vi "USRP Throughput Streaming (FPGA).vi"() -> ()   [LabVIEW 2016]
doc: "Example Description:\nThis FPGA VI has two data streaming engines. One to stream data to disk from the FPGA and one to stream data from disk to the FPGA. The throughput of the streams is controled by accessing the DMA FIFOs on a subset of the cycles of the SCTLs.\n\nRunning the VI:\nThis VI m ust be run from one of the High Throughput Streaming - XXXXXXX (Host).vi files in the project. Refer to the host documentation for steps regarding running and configuring this FPGA VI.\n\nExecution Steps:\nRefer to teh block diagram of this VI for excution comments."
uses:
  <instrlib>/_niInstr/Register Bus/v1/FPGA/Public/Read Cmd Data.ctl
  <vilib>/Platform/TimedLoop/XDataNode/timing_clust.ctl
  <vilib>/Platform/TimedLoop/XDataNode/nitl_modes.ctl
  <vilib>/Platform/TimedLoop/XDataNode/wakeup.ctl
  <vilib>/rvi/Emulation/niFpgaSctlEmulationGetInTimedLoop.vi
  <vilib>/rvi/Emulation/niFpgaEmulationReportErrorSimple.vi
  <vilib>/rvi/Emulation/niFpgaGetClockAttributes.vi
  <vilib>/rvi/Emulation/niFpgaCriticalErrorInLSC.vi
  <vilib>/rvi/interface/RandomDataEmulation/nirviRandomDataMultiElementFPGAFIFO.vi
  <instcachedir>/0/nirviRandomDataMultiElementFPGAFIFO_6740B454F3C245F78F76ED91F73FD8DB.lvgen/nirviRandomDataMultiElementFPGAFIFO_6740B454F3C245F78F76ED91F73FD8DB_004.vi
  <vilib>/rvi/interface/RandomDataEmulation/niFpgaRandomDataHandleErrors.vi
  <vilib>/rvi/eio/common/nirviEmuTemplateMethod_errors.vi
  <vilib>/Platform/TimedLoop/XDataNode/XDataNode.xnode
  <vilib>/rvi/DataTransferAndStorage/Container/XNode/niFpgaContainer.xnode
  <vilib>/rvi/interface/RandomDataEmulation/nirviRandomDataFpgaMultiElementTemplate.vi
  <vilib>/eio/EIONode/EIONode.xnode
  <vilib>/Platform/TimedLoop/XDataNode/XDNodeRunTimeDep.lvlib
  <instrlib>/_niInstr/Register Bus/v1/FPGA/niInstr Register Bus v1 FPGA.lvlib
  <instrlib>/niUsrpRio/Config/v1/FPGA/niUsrpRio Config v1 FPGA.lvlib
panel:
  out "input.Max Throughput":u16
  out "output.Max Throughput":u16
  out "output.FIFO Size":u32
  out "input.FIFO Size":u32
  out "output.Ever Timed Out?":bool
  in  "output.Reset":bool
  out "output.Number of Elements to Read":u32
  out "output.Minimum Number of Elements to Read":u32
  out "output.FIFO Transfer Status":T1
  in  "output.Requested Throughput":u16
  in  "output.Requested Throughput Denominator":u16=200
  out "input.Ever Timed Out?":bool
  in  "input.Reset":bool
  out "input.Number of Elements to Write":u32
  out "input.Minimum Number of Elements to Write":u32
  out "input.FIFO Transfer Status":T2
  in  "input.Requested Throughput":u16
  in  "input.Requested Throughput Denominator":u16=200
  in  "reg.host read.go rcvd 0":bool
  out "reg.notify host.go 0":bool
  in  "reg.notify host.go rcvd 0":bool
  out "reg.host read.data 0":T3
  in  "reg.reset 0":bool
  in  "RF 0/Rx/Enable":bool
  in  "RF 0/Tx/Enable":bool
  in  "RF 1/Rx/Enable":bool
  in  "RF 1/Tx/Enable":bool
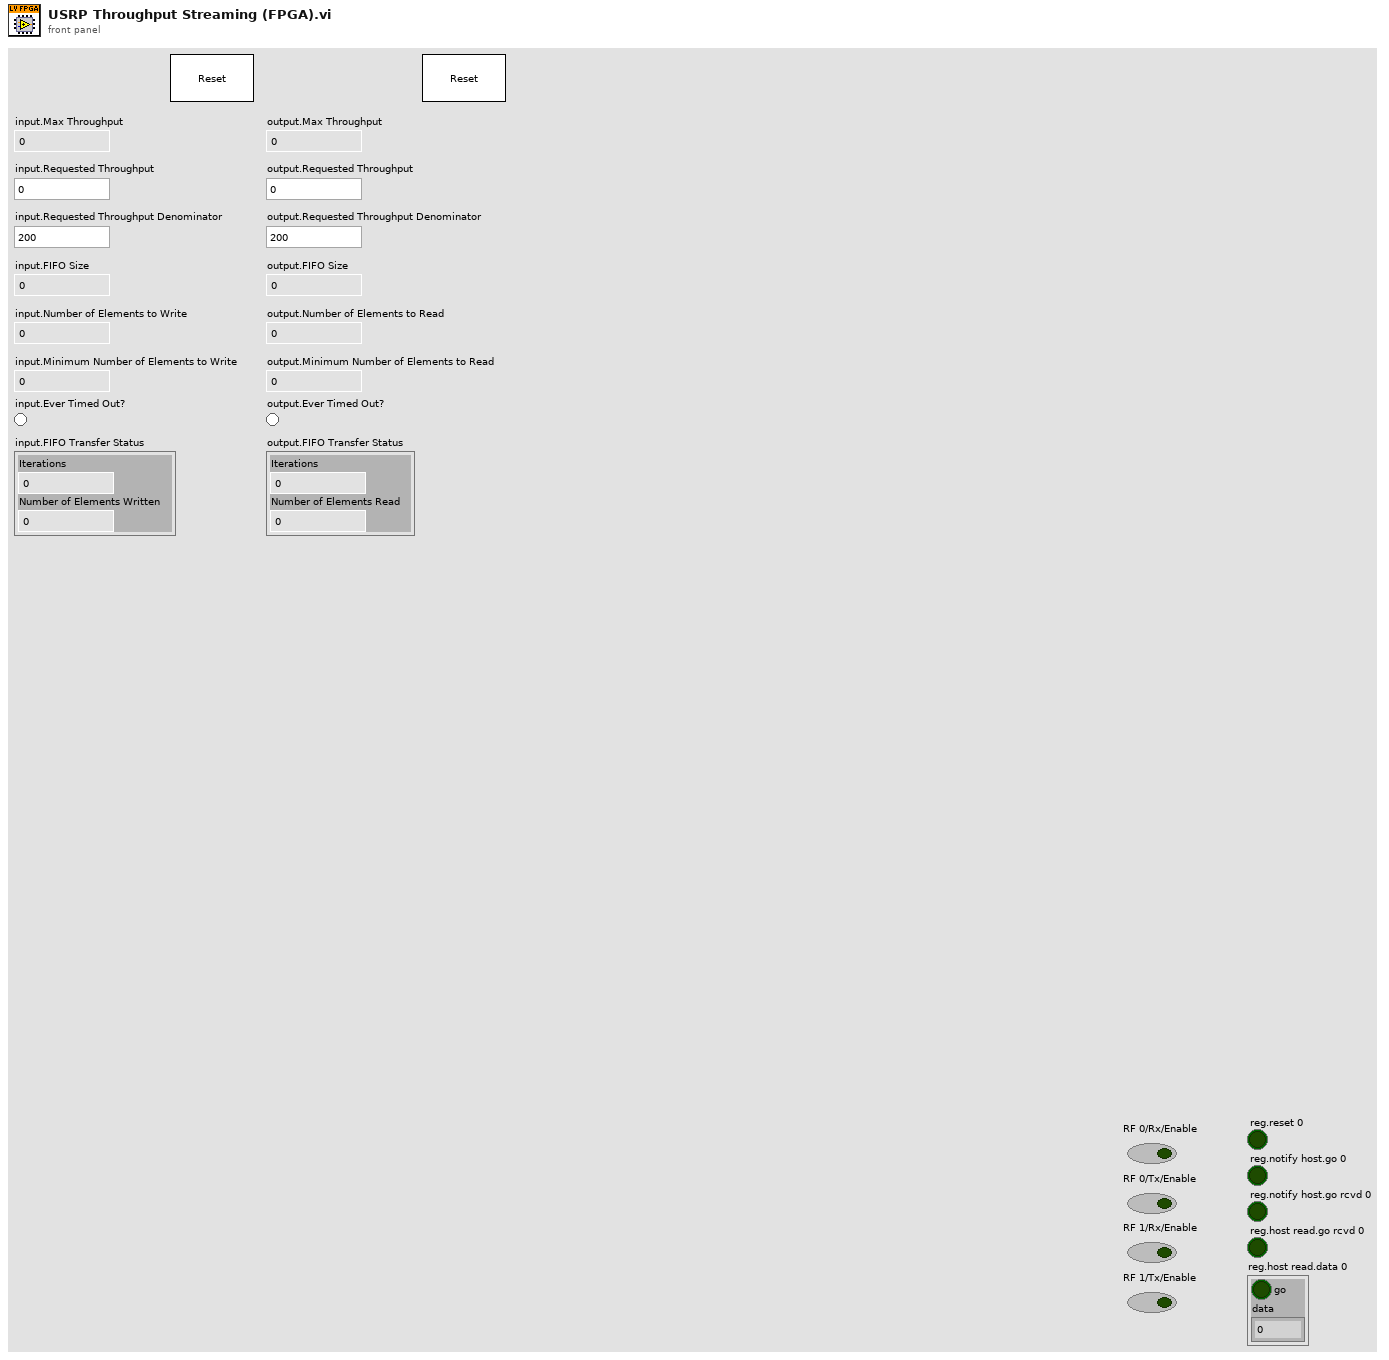
[diagram p1: front panel]
types:
  T1 = cluster{"Iterations":u64, "Number of Elements Read":u64}
  T2 = cluster{"Iterations":u64, "Number of Elements Written":u64}
  T3 = typedef "niInstr Register Bus v1 FPGA.lvlib/Read Cmd Data.ctl" = cluster{"go":bool, "data":u32}
  T4 = typedef "XDNodeRunTimeDep.lvlib/timing_clust.ctl" = cluster{"Expected End [f-1]":u64, "Actual End [f-1]":u64, "Finished Late? [f-1]":bool, "Expected End [i-1]":u64, "Actual End [i-1]":u64, "Finished Late? [i-1]":bool, "Expected Start [i]":u64, "Actual Start [i]":u64, "Expected Start [f]":u64, "Actual Start [f]":u64, "Source Name":string, "Structure Name":string, "Period":i64, "Deadline":i64, "Offset":i64, "Start":i64, "Priority":i32, "Timeout":i32, "Mode":T5, "Wakeup Reason":T6, "Error":errorcluster, "Source Type":string, "Secondary Source Type":string, "Global End Time":u64, "Global Start Time":u64, "Frame Duration":u64, "Iteration Duration":u64, "Assigned CPU":i32, "I/O Scan Engine Mode":u32}
  T5 = typedef "XDNodeRunTimeDep.lvlib/nitl_modes.ctl" = enum32{"No Change", "Process missed periods, maintain original phase", "Discard missed periods, maintain original phase", "Process missed periods, ignore original phase", "Discard missed periods, ignore original phase"}
  T6 = typedef "XDNodeRunTimeDep.lvlib/wakeup.ctl" = enum32{"Normal", "Aborted", "Asynchronous wakeup", "Timing source error", "Timed loop error", "Timeout"}
  T7 = cluster{"DAC FIFO Reset":refnum<k21>, "RF 0 Rx Swap IQ":refnum<k21>, "RF 0 Rx Negate I":refnum<k21>, "RF 0 Rx Negate Q":refnum<k21>, "RF 0 Rx Data Valid":refnum<k21>, "RF 0 Rx Data Ever Invalid":refnum<k21>, "clear RF 0 Rx Data Ever Invalid":refnum<k21>, "RF 0 Tx Swap IQ":refnum<k21>, "RF 0 Tx Negate I":refnum<k21>, "RF 0 Tx Negate Q":refnum<k21>, "RF 1 Rx Swap IQ":refnum<k21>, "RF 1 Rx Negate I":refnum<k21>, "RF 1 Rx Negate Q":refnum<k21>, "RF 1 Rx Data Valid":refnum<k21>, "RF 1 Rx Data Ever Invalid":refnum<k21>, "clear RF 1 Rx Data Ever Invalid":refnum<k21>, "RF 1 Tx Swap IQ":refnum<k21>, "RF 1 Tx Negate I":refnum<k21>, "RF 1 Tx Negate Q":refnum<k21>}
  T8 = typedef "niUsrpRio Synchronization v1 FPGA.lvlib/Resources.ctl" = cluster{"master":refnum<k21>, "meas.enable":refnum<k21>, "meas.ready":refnum<k21>, "meas.reset":refnum<k21>, "meas.arm":refnum<k21>, "meas.valid":refnum<k21>, "meas.value":refnum<k21>, "meas.oversample factor":refnum<k21>, "cptr":refnum<k21>, "cptr.adjust":refnum<k21>, "cptr.period":refnum<k21>}
  T9 = typedef "niUsrpRio Time v1 FPGA.lvlib/Time Resources.ctl" = cluster{"reset":refnum<k21>, "time":refnum<k21>, "time.previous cptr":refnum<k21>, "new time":refnum<k21>, "new time.when":refnum<k21>, "new time.set":refnum<k21>, "which edge of ref":refnum<k21>, "pps source":refnum<k21>, "internal pps period":refnum<k21>}
  T10 = typedef "niUsrpRio Time v1 FPGA.lvlib/Future Event Resources.ctl" = cluster{"reset":refnum<k21>, "future event.time":refnum<k21>, "future event.ready":refnum<k21>, "future event.set":refnum<k21>, "future event.clear":refnum<k21>, "future event.set in past":refnum<k21>}
  T11 = cluster{"time.resources":T9, "future event.resources":T10, "future event.resources":T10, "future event.resources":T10}
  T12 = typedef "niInstr Register Bus v1 FPGA.lvlib/Register Instruction.ctl" = cluster{"subsystem":u8, "address":u16, "data":u32, "valid":bool, "read":bool}
  T13 = typedef "niInstr Register Bus v1 FPGA.lvlib/Read Completion.ctl" = cluster{"data":u32, "valid":bool}
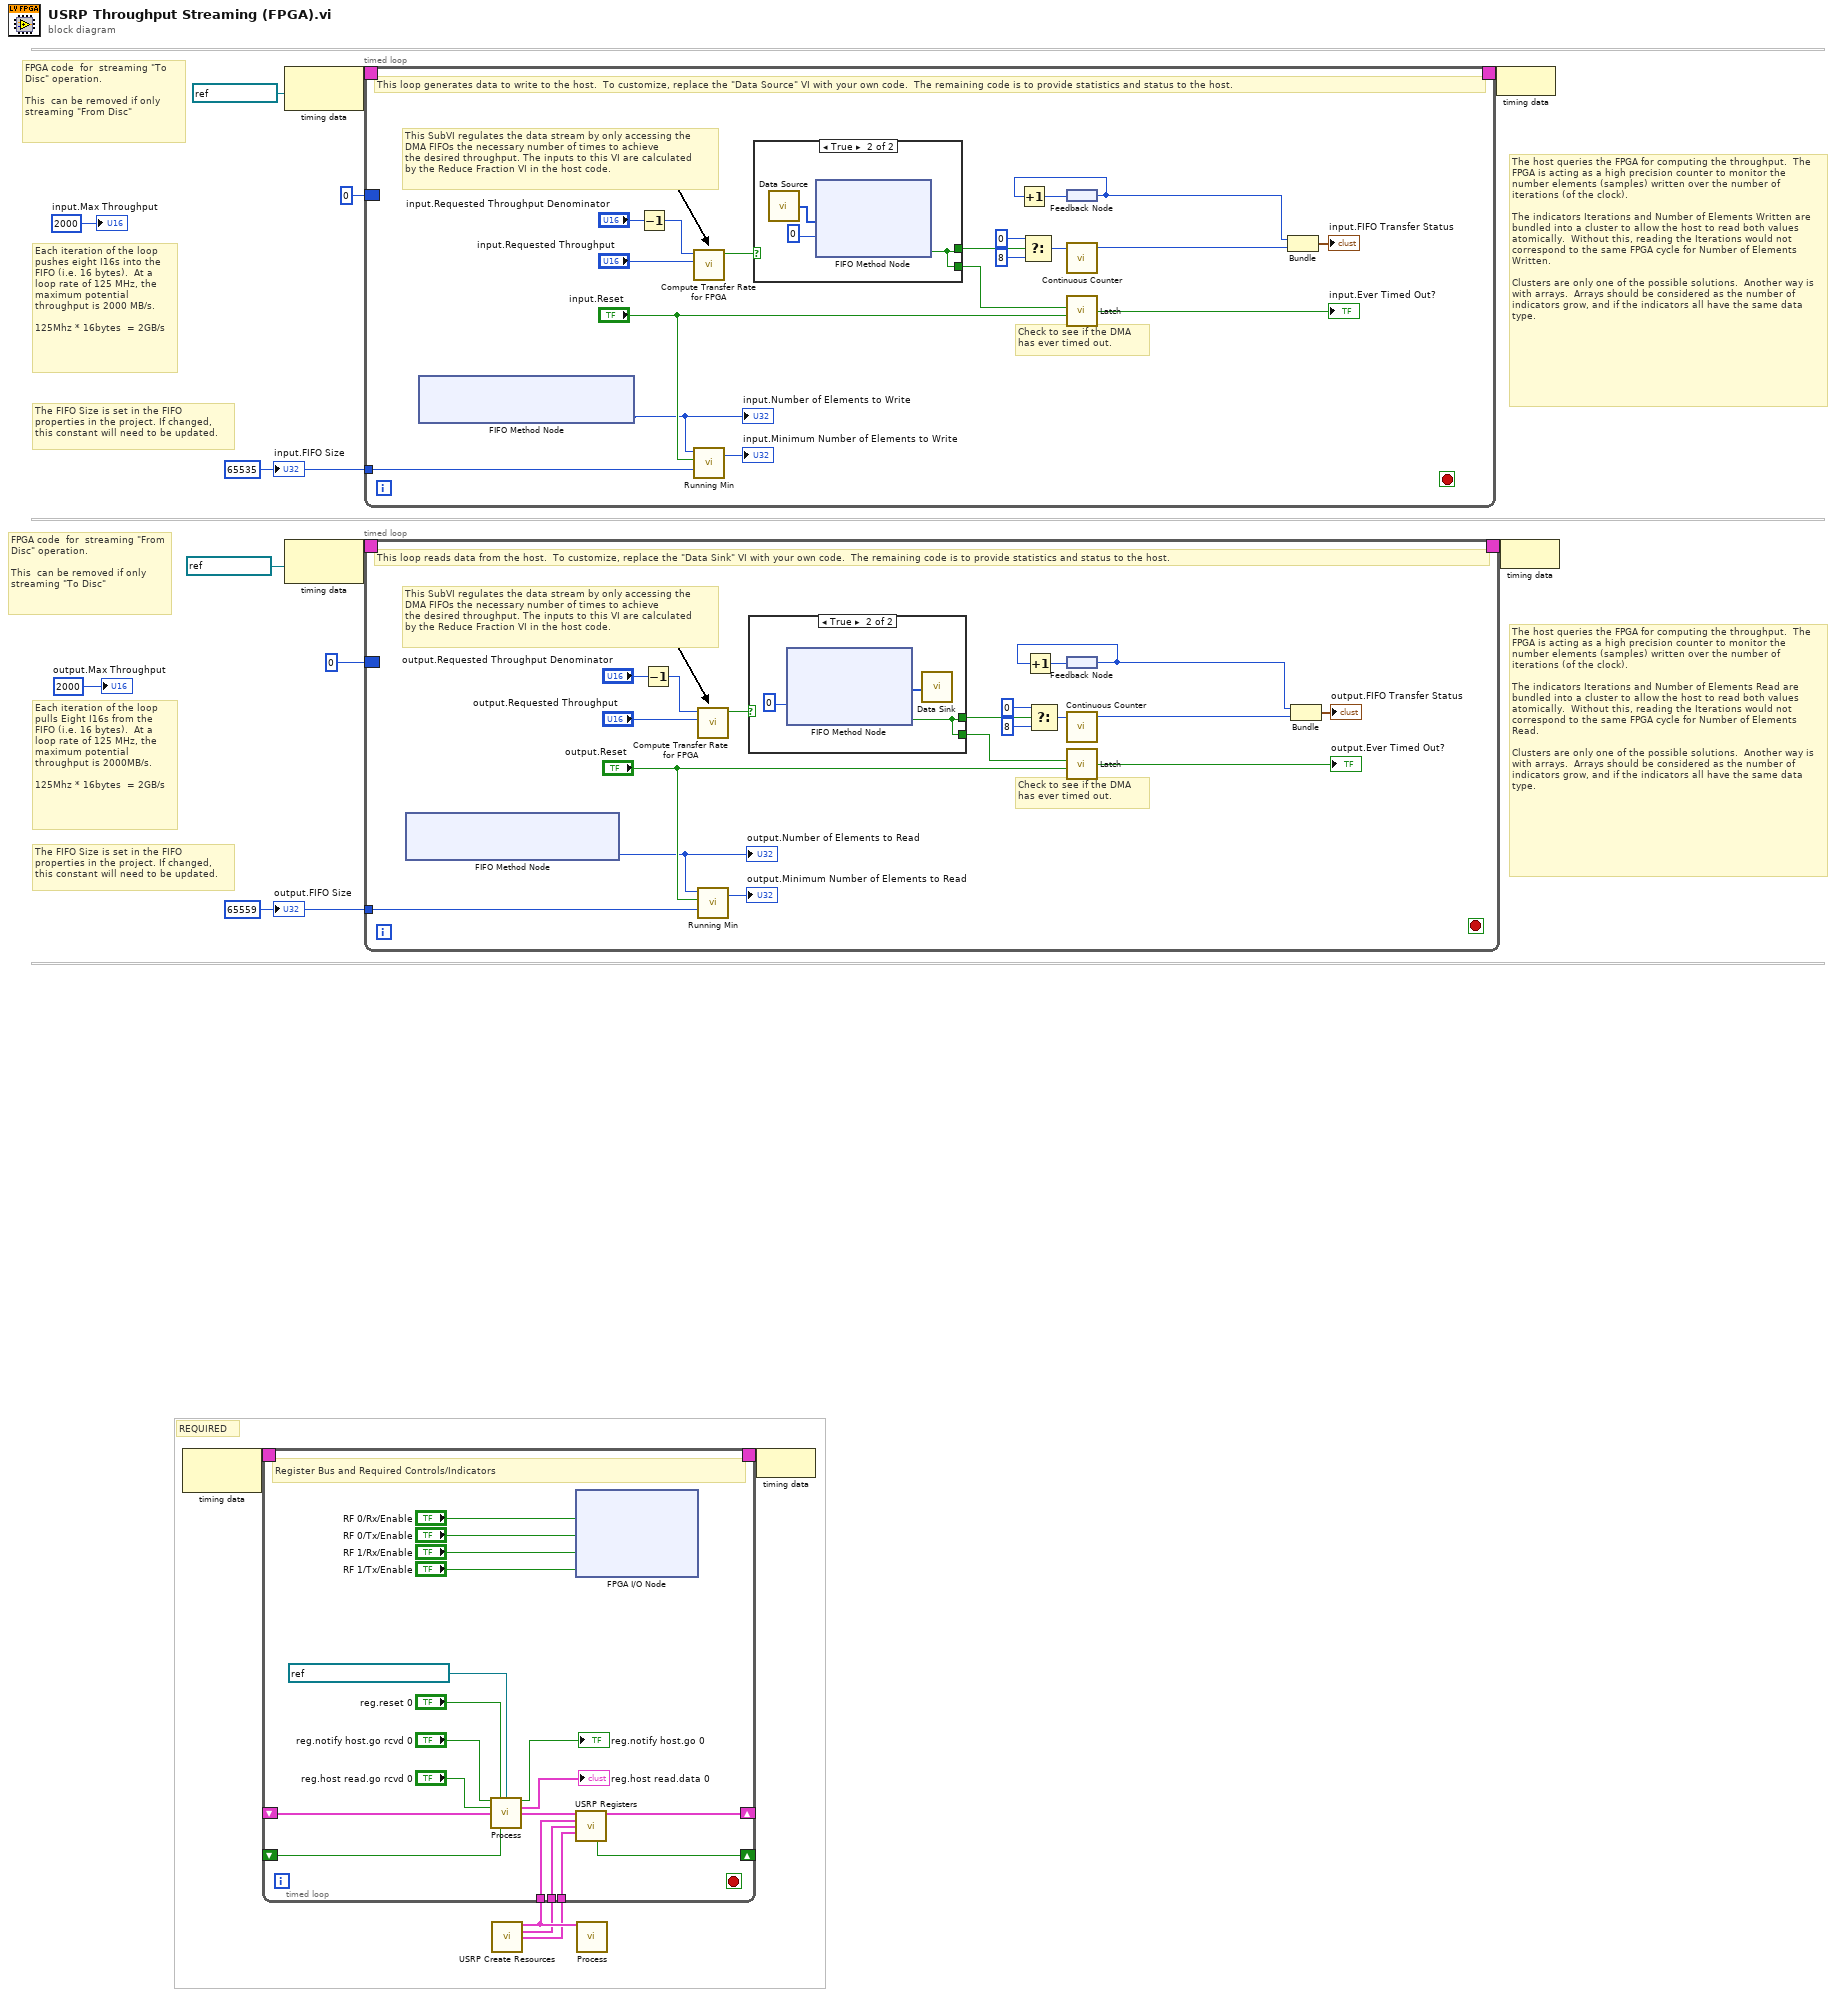
[diagram p0: block diagram]
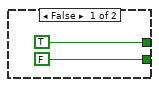
[diagram p2: hidden frame]
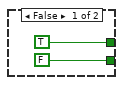
[diagram p3: hidden frame]
diagram:
  w6 = u32 65559 ("output.FIFO Size")
  w3 = u32 65535 ("input.FIFO Size")
  # "The FIFO Size is set in the FIFO\nproperties in the project. If changed, \nthis constant will need to be updated."
  # "The FIFO Size is set in the FIFO\nproperties in the project. If changed, \nthis constant will need to be updated."
  # "FPGA code  for  streaming \"To Disc\" operation. \n\nThis  can be removed if only streaming \"From Disc\""
  # "FPGA code  for  streaming \"From Disc\" operation. \n\nThis  can be removed if only streaming \"To Disc\""
  # "Each iteration of the loop pulls Eight I16s from the FIFO (i.e. 16 bytes).  At a loop rate of 125 MHz, the maximum potential throughput is 2000MB/s.\n\n125Mhz * 16bytes  = 2GB/s"
  # "The host queries the FPGA for computing the throughput.  The FPGA is acting as a high precision counter to monitor the number elements (samples) written over the number of iterations (of the clock).\n\nThe indicators Iterations and Number of Elements Read are bundled into a cluster to allow the host to read both values atomically.  Without this, reading the Iterations would not correspond to the same FPGA cycle for Number of Elements Read.\n\nClusters are only one of the possible solutions.  Another way is with arrays.  Arrays should be considered as the number of indicators grow, and if the indicators all have the same data type."
  # "Each iteration of the loop pushes eight I16s into the FIFO (i.e. 16 bytes).  At a loop rate of 125 MHz, the maximum potential throughput is 2000 MB/s.\n\n125Mhz * 16bytes  = 2GB/s"
  # "The host queries the FPGA for computing the throughput.  The FPGA is acting as a high precision counter to monitor the number elements (samples) written over the number of iterations (of the clock).\n\nThe indicators Iterations and Number of Elements Written are bundled into a cluster to allow the host to read both values atomically.  Without this, reading the Iterations would not correspond to the same FPGA cycle for Number of Elements Written.\n\nClusters are only one of the possible solutions.  Another way is with arrays.  Arrays should be considered as the number of indicators grow, and if the indicators all have the same data type."
  # "REQUIRED"
  n1 = node-c288() -> (w17:T4)  [unwired: 1 in]
  n2 = node-c288(refnum<k21> "Data Clock" ("Source Name")) -> (w12:T4)
  n3 = node-c288(refnum<k21> "Data Clock" ("Source Name")) -> (w10:T4)
  n4 = timed-loop {
    timing: w12 -> [_]
    timing-out: [_] -> w11
    tunnel: w3 -> [w35]
    border: u64 0 -> [_]
    stop <- _ stop-if-true
    # "Check to see if the DMA \nhas ever timed out."
    # "This SubVI regulates the data stream by only accessing the \nDMA FIFOs the necessary number of times to achieve \nthe desired throughput. The inputs to this VI are calculated \nby the Reduce Fraction VI in the host code."
    # "This loop generates data to write to the host.  To customize, replace the \"Data Source\" VI with your own code.  The remaining code is to provide statistics and status to the host."
    n5 = xnode ("FIFO Method Node")() -> ("Number of Elements to Write"=w18:u32)  [unwired: 1 in, 1 out]
    "input.Number of Elements to Write" <- w18
    n6 = Decrement(x="input.Requested Throughput Denominator") -> (x-1=w20:u16)
    n7 = call "Compute Transfer Rate for FPGA.vi"("Duty Rate"="input.Requested Throughput", "Clock Rate (minus 1)"=w20) -> ("Output"=w23:bool)  [unwired: 4 in, 1 out]
    n8 = call "Running Min.vi"("Starting Min"=w35, "Reset"="input.Reset", "Next Value"=w18) -> ("Running Min"=→"input.Minimum Number of Elements to Write":u32)  [unwired: 4 in]
    n9 = case shown="True" w23 {
      tunnel: [TRUE ("Timed Out?") w38] -> w22
      tunnel: [FALSE ("Timed Out?") w38] -> w21
      frame False {
      }
      frame True {
        n10 = call "Data Source.vi"() -> ("Elements"=w40:i16[])
        n11 = xnode ("FIFO Method Node")("Element"=w40, "Timeout"=0) -> ("Timed Out?"=w38:bool)  [unwired: 1 in, 1 out]
      }
    }
    n12 = Select(t=u8 0, s=w22, f=u8 8) -> (s? t:f=w31:u8)
    n13 = feedback #1() -> (w28:u64)
    n14 = Increment(x=w28) -> (x+1=w29:u64)
    n15 = feedback-in #1(w29) -> ()
    n16 = call "Continuous Counter.vi"("value"=w31) -> ("count"=w27:u64)  [unwired: 6 in]
    n17 = call <vilib>:"Latch.vi"("Clear"="input.Reset", "Set"=w21) -> ("Output"=→"input.Ever Timed Out?":bool)  [unwired: 4 in]
    n18 = Bundle(w28, "count"=w27) -> (→"input.FIFO Transfer Status":cluster{u64, "count":u64})  [unwired: 1 in]
  }
  n19 = timed-loop {
    timing: w10 -> [_]
    timing-out: [_] -> w9
    border: u64 0 -> [_]
    tunnel: w6 -> [w52]
    stop <- _ stop-if-true
    # "Check to see if the DMA \nhas ever timed out."
    # "This SubVI regulates the data stream by only accessing the \nDMA FIFOs the necessary number of times to achieve \nthe desired throughput. The inputs to this VI are calculated \nby the Reduce Fraction VI in the host code."
    # "This loop reads data from the host.  To customize, replace the \"Data Sink\" VI with your own code.  The remaining code is to provide statistics and status to the host."
    n20 = xnode ("FIFO Method Node")() -> ("Number of Elements to Read"=w43:u32)  [unwired: 1 in, 1 out]
    "output.Number of Elements to Read" <- w43
    n21 = Decrement(x="output.Requested Throughput Denominator") -> (x-1=w45:u16)
    n22 = call "Compute Transfer Rate for FPGA.vi"("Duty Rate"="output.Requested Throughput", "Clock Rate (minus 1)"=w45) -> ("Output"=w48:bool)  [unwired: 4 in, 1 out]
    n23 = call "Running Min.vi"("Starting Min"=w52, "Reset"="output.Reset", "Next Value"=w43) -> ("Running Min"=→"output.Minimum Number of Elements to Read":u32)  [unwired: 4 in]
    n24 = case shown="True" w48 {
      tunnel: [TRUE ("Timed Out?") w63] -> w54
      tunnel: [FALSE ("Timed Out?") w63] -> w46
      frame False {
      }
      frame True {
        n25 = xnode ("FIFO Method Node")("Timeout"=0) -> ("Element"=w64:i16[], "Timed Out?"=w63:bool)  [unwired: 1 in, 1 out]
        n26 = call "Data Sink.vi"("Elements"=w64) -> ()
      }
    }
    n27 = Select(t=u8 0, s=w54, f=u8 8) -> (s? t:f=w57:u8)
    n28 = feedback #2() -> (w51:u64)
    n29 = Increment(x=w51) -> (x+1=w59:u64)
    n30 = feedback-in #2(w59) -> ()
    n31 = call "Continuous Counter.vi"("value"=w57) -> ("count"=w50:u64)  [unwired: 6 in]
    n32 = call <vilib>:"Latch.vi"("Clear"="output.Reset", "Set"=w46) -> ("Output"=→"output.Ever Timed Out?":bool)  [unwired: 4 in]
    n33 = Bundle(w51, "count"=w50) -> (→"output.FIFO Transfer Status":cluster{u64, "count":u64})  [unwired: 1 in]
  }
  n34 = call "USRP Create Resources.vi"() -> ("config.resources"=w15:T7, "sync.resources"=w14:T8, "time.resources"=w13:T11)  [unwired: 13 in]
  n35 = timed-loop "Register Bus and Required Controls/Indicators" {
    timing: w17 -> [_]
    timing-out: [_] -> w16
    shift-right: [w82] -> _
    shift-left: _ -> [w81]
    shift-right: [w76] -> _
    shift-left: _ -> [w80]
    tunnel: w15 -> [w74]
    tunnel: w14 -> [w73]
    tunnel: w13 -> [w72]
    stop <- _ stop-if-true
    # "Register Bus and Required Controls/Indicators"
    n36 = call <instrlib>:"Process.vi"("reg.notify host.go rcvd"="reg.notify host.go rcvd 0", "reg.reset"="reg.reset 0", "reg.host instruction fifo"=refnum<k21> "reg.host instruction fifo 0", "reg.host read.go rcvd"="reg.host read.go rcvd 0", "read completion"=w81, "ready for output"=w80) -> ("reg.notify host.go"=→"reg.notify host.go 0":bool, "reg.host read.data"=→"reg.host read.data 0":T3, "register instruction"=w75:T12)  [unwired: 7 in]
    n37 = xnode ("FPGA I/O Node")("RF 0/Rx/Enable"="RF 0/Rx/Enable", "RF 0/Tx/Enable"="RF 0/Tx/Enable", "RF 1/Rx/Enable"="RF 1/Rx/Enable", "RF 1/Tx/Enable"="RF 1/Tx/Enable") -> ()  [unwired: 4 in, 4 out]
    n38 = call "USRP Registers.vi"("register instruction"=w75, "config.resources"=w74, "sync.resources"=w73, "time.resources"=w72) -> ("read completion out"=w82:T13, "ready for input"=w76:bool)  [unwired: 10 in]
  }
  n39 = call <instrlib>:"Process.vi"("resources"=w15) -> ()  [unwired: 15 in]
  n40 = node-c288(w16) -> ()
  n41 = node-c288(w11) -> ()
  n42 = node-c288(w9) -> ()
  "input.FIFO Size" <- w3
  "output.FIFO Size" <- w6
  "output.Max Throughput" <- u16 2000 ("output.Max Throughput")
  "input.Max Throughput" <- u16 2000 ("input.Max Throughput")
